vi "LoadUserInterface.vi"(8 "error in (no error)":errorcluster, 10 "Actor In":refnum<class "Actor.lvclass">, 11 "DataProcessor in":refnum<class "DataProcessor.lvclass">) -> (0 "error out":errorcluster, 3 "DataProcessor out":refnum<class "DataProcessor.lvclass">)   [LabVIEW 2020, in "DataProcessor.lvlib" / "DataProcessor.lvclass"]
uses:
  DataProcessor.lvclass
  C:/Program Files/National Instruments/LabVIEW 2020/vi.lib/ActorFramework/Actor/Actor.lvclass
  <vilib>/ActorFramework/Actor/Actor.lvclass
  DataProcessor.lvclass/DataProcessor.ctl
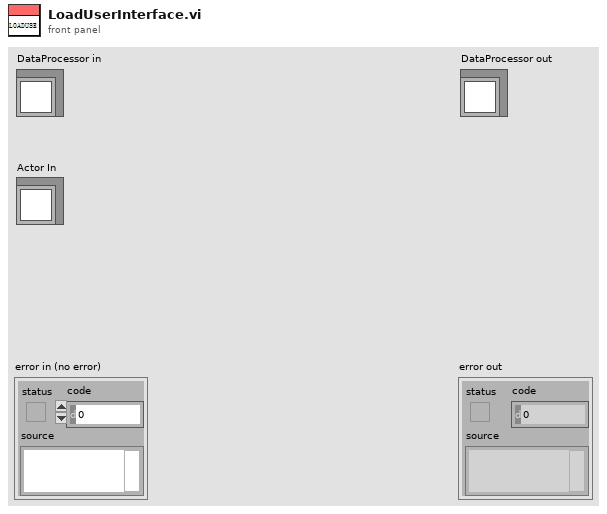
[diagram p1: front panel]
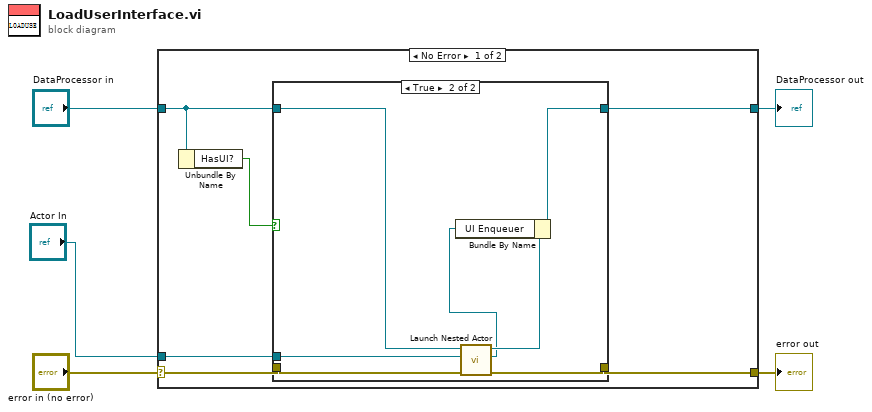
[diagram p0: block diagram]
diagram:
  n1 = case shown="No Error" "error in (no error)" {
    selector: "error in (no error)" -> [w11 w22]
    tunnel: [w10 w22] -> w4
    tunnel: [w8 w21] -> w2
    tunnel: "DataProcessor in" -> [w7 w21]
    tunnel: "Actor In" -> [w9 _]
    frame No Error {
      n2 = Unbundle By Name(w7) -> ("HasUI?"=w6:bool)
      n3 = case shown="True" w6 {
        tunnel: w11 -> [w12 w20]
        tunnel: [w12 w19] -> w10
        tunnel: w7 -> [w13 w18]
        tunnel: w9 -> [_ w16]
        tunnel: [w13 w15] -> w8
        frame False {
        }
        frame True {
          n4 = call <vilib>:"Launch Nested Actor.vi"("error in (no error)"=w20, "Nested Actor"=w16, "Caller Actor in"=w18) -> ("error out"=w19:errorcluster, "Nested Actor's Enqueuer"=w14:refnum<class "Message Enqueuer.lvclass">, "Caller Actor out"=w17:refnum<class "DataProcessor.lvclass">)  [unwired: 6 in]
          n5 = Bundle By Name(cluster=w17, "UI Enqueuer"=w14) -> (w15:refnum<class "DataProcessor.lvclass">)
        }
      }
    }
    frame Error {
    }
  }
  "error out" <- w4
  "DataProcessor out" <- w2
